vi "DigitalINTriggerSet.vi"(4 "Fall":u32 format="%.0x", 5 "timeout":i32, 6 "Rais":u32 format="%.0x", 7 "trigcond":enum16{"Raising", "Falling", "Either"}(ring), 8 "error in (no error)":errorcluster caption="错误输入（无错误）", 9 "trigtype":enum16{"edge", "pulse", "trasition"}(ring), 10 "trigsrc":T1(ring), 11 "handle":u64) -> (0 "error out":errorcluster caption="错误输出", 2 "function return":i32, 3 "handle out":u64)   [LabVIEW 2018]
doc: "Set pos. or neg. Supply voltage"
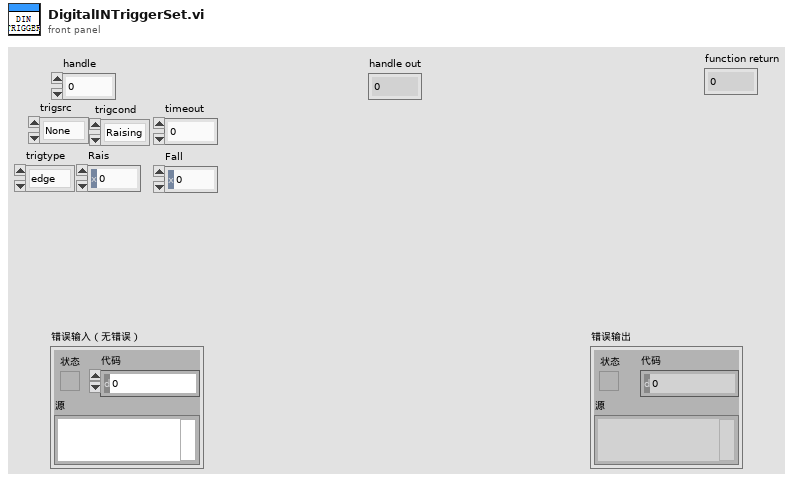
[diagram p1: front panel]
types:
  T1 = enum16{"None", "DetectorAnalogInCH1", "DetectorAnalogInCH2", "AnalogOut1", "AnalogOut2", "DetectorDigitalIn", "DigitalOut", "Manule", "External 1", "External 2", "DigitalIn"}
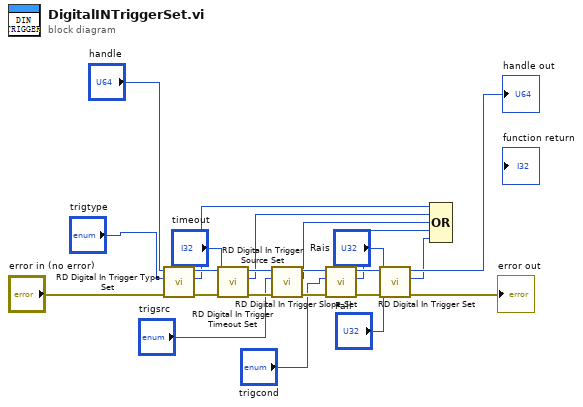
[diagram p0: block diagram]
diagram:
  n1 = call "RD Digital In Trigger Type Set.vi"("error in (no error)"="error in (no error)", "type"="trigtype", "handle"="handle") -> ("error out"=w13:errorcluster, "function return"=w11:i32, "handle out"=w19:u64)  [unwired: 6 in]
  n2 = call "RD Digital In Trigger Timeout Set.vi"("error in (no error)"=w13, "enable"="timeout", "handle"=w19) -> ("error out"=w14:errorcluster, "function return"=w10:i32, "handle out"=w20:u64)  [unwired: 6 in]
  n3 = call "RD Digital In Trigger Source Set.vi"("error in (no error)"=w14, "trigsrc"="trigsrc", "handle"=w20) -> ("error out"=w16:errorcluster, "function return"=w9:i32, "handle out"=w21:u64)  [unwired: 6 in]
  n4 = call "RD Digital In Trigger Slope Set.vi"("error in (no error)"=w16, "slope"="trigcond", "handle"=w21) -> ("error out"=w17:errorcluster, "function return"=w8:i32, "handle out"=w22:u64)  [unwired: 6 in]
  n5 = call "RD Digital In Trigger Set.vi"("error in (no error)"=w17, "Fall"="Fall", "Rais"="Rais", "handle"=w22) -> ("error out"=→"error out":errorcluster, "function return"=w7:i32, "handle out"=→"handle out":u64)  [unwired: 5 in]
  n6 = Compound Arithmetic op=OR ("复合运算")(w11, w10, w9, w8, w7) -> ()  [unwired: 1 out]
